vi "MACBIN Has Resource Fork__ogtk.vi"(4 "error in (no error)":errorcluster, 7 "file path":path) -> (0 "error out":errorcluster, 2 "has resource fork":bool, 3 "file path out":path)   [LabVIEW 2020]
doc: "Checks if a Macintosh file has a resource fork. NOP on non Macintosh systems."
uses:
  <userlib>/_OpenG.lib/lvzip/lvzlib.dll
panel:
  # "Please visit http://www.OpenG.org to learn about the\nOpen Source LabVIEW software movement.\n\nNOTICE -- YOU MUST LEAVE THIS NOTICE IN PLACE.  PER THE TERMS OF THE LICENSE BELOW, YOU MAY SUBLICENSE THIS SOFTWARE \nIN ANY WAY THAT DOES NOT CONFLICT WITH THIS LICENSE.\n\n### BSD License (http://www.opensource.org/licenses/bsd-license.php) Begin ###\n \nCopyright (C) 2002 Christophe Salzmann christophe.salzmann@epfl.ch\nCopyright (C) 2002-2006 Rolf Kalbermatter rolf.kalbermatter@citengineering.com\n\nAll rights reserved.\n\nRedistribution and use in source and binary forms, with or without modification, are permitted provided that the following conditions are met:\n\n    * Redistributions of source code must retain the above copyright notice, this list of conditions and the following disclaimer.\n    * Redistributions in binary form must reproduce the above copyright notice, this list of conditions and the following disclaimer in the \n       documentation and/or other materials provided with the distribution.\n    * Neither the name of SciWare, James Kring, Inc., nor the names of its contributors may be used to endorse or promote products derived \n       from this software without specific prior written permission.\n\nTHIS SOFTWARE IS PROVIDED BY THE COPYRIGHT HOLDERS AND CONTRIBUTORS \"AS IS\" AND ANY EXPRESS OR IMPLIED WARRANTIES, \nINCLUDING, BUT NOT LIMITED TO, THE IMPLIED WARRANTIES OF MERCHANTABILITY AND FITNESS FOR A PARTICULAR PURPOSE ARE \nDISCLAIMED. IN NO EVENT SHALL THE COPYRIGHT OWNER OR CONTRIBUTORS BE LIABLE FOR ANY DIRECT, INDIRECT, INCIDENTAL,\n SPECIAL, EXEMPLARY, OR CONSEQUENTIAL DAMAGES (INCLUDING, BUT NOT LIMITED TO, PROCUREMENT OF SUBSTITUTE GOODS OR \nSERVICES; LOSS OF USE, DATA, OR PROFITS; OR BUSINESS INTERRUPTION) HOWEVER CAUSED AND ON ANY THEORY OF LIABILITY, \nWHETHER IN CONTRACT, STRICT LIABILITY, OR TORT (INCLUDING NEGLIGENCE OR OTHERWISE) ARISING IN ANY WAY OUT OF THE USE \nOF THIS SOFTWARE, EVEN IF ADVISED OF THE POSSIBILITY OF SUCH DAMAGE.\n\n### BSD License End ###"
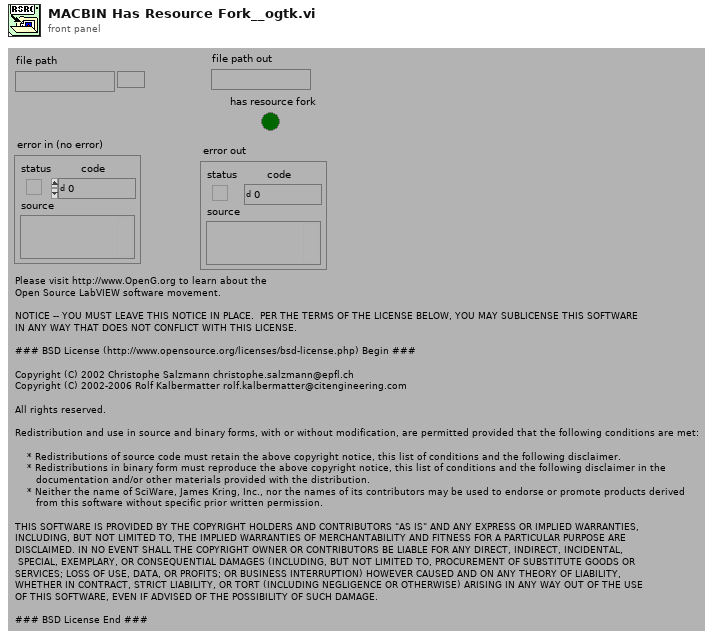
[diagram p1: front panel]
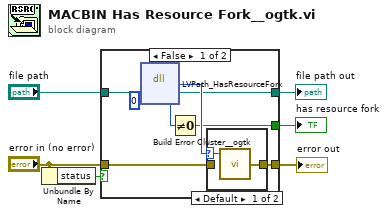
[diagram p0: block diagram]
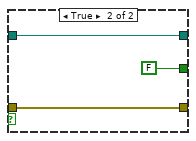
[diagram p3: hidden frame]
diagram:
  n1 = Unbundle By Name("error in (no error)") -> ("status"=w6:bool)
  n2 = case shown="False" w6 {
    tunnel: "file path" -> [w8 w18]
    tunnel: "error in (no error)" -> [w14 w20]
    tunnel: [w13 w20] -> w4
    tunnel: [w10 FALSE] -> w3
    tunnel: [w7 w18] -> w2
    frame False {
      n3 = dll-call lib="D:/Projects/OpenG/opengtoolkit/lvzip/source/lvzlib.*" fn="LVPath_HasResourceFork"("file path"=w8, "hasRsrc"=0) -> (w12:i32, "file path"=w7:path, "hasRsrc"=w9:i32)  [unwired: 3 in, 2 out]
      n4 = Not Equal To 0?(x=w9) -> (x != 0?=w10:bool)
      n5 = case shown="Default" w12 {
        selector: w12 -> [w16 _]
        tunnel: w14 -> [_ w17]
        tunnel: [w15 w17] -> w13
        frame Default {
          n6 = call <userlib>:"Build Error Cluster__ogtk.vi"("code"=w16) -> ("error out"=w15:errorcluster)  [unwired: 1 in]
        }
        frame 0 {
        }
      }
    }
    frame True {
    }
  }
  "error out" <- w4
  "has resource fork" <- w3
  "file path out" <- w2
